vi "测试中.vi"(6 "测试数据":dbl[][](array[numeric]), 7 "XY图":refnum<vi>, 8 "曲线设置":T1={"X轴数据选择"=enum."设置电压", "Y轴组"=[]}, 10 "错误输入（无错误）":errorcluster) -> (2 "错误输出":errorcluster)   [LabVIEW 2021]
uses:
  <vilib>/Utility/miscctls.llb/LVCursorListTypeDef.ctl
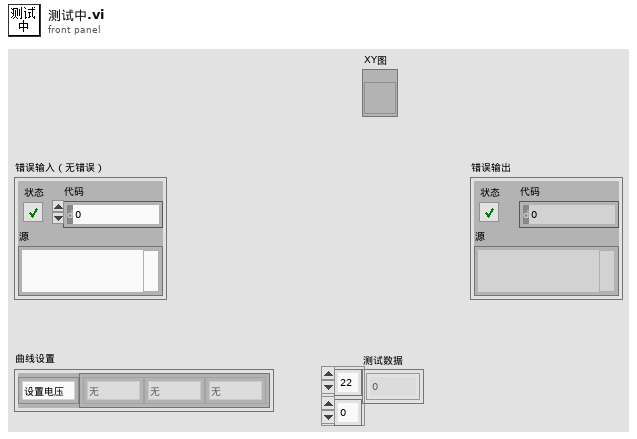
[diagram p1: front panel]
types:
  T1 = typedef "曲线设置.ctl" = cluster{"X轴数据选择":enum16{"时间", "设置电压", "读取电流", "读取电压"}, "Y轴组":enum16{"时间", "设置电压", "读取电流", "读取电压", "无"}[]}
  T2 = typedef "LVCursorListTypeDef.ctl" = cluster{"Name":string, "Color":u32, "Style":u8, "Point Style":u8, "Name Visible":bool, "Allow Drag":bool, "Cursor Mode":u32, "Plot":i32, "Index":i32, "Position":cluster{"X":dbl, "Y":dbl}, "X Scale":u32, "Y Scale":u32, "Watch Plots":i32[], "Watch All Plots":bool, "Plot Area":i32, "Label Offset":cluster{"X":dbl, "Y":dbl}}[]
  T3 = typedef "曲线属性.ctl" = cluster{"曲线名":string, "曲线颜色":u32}
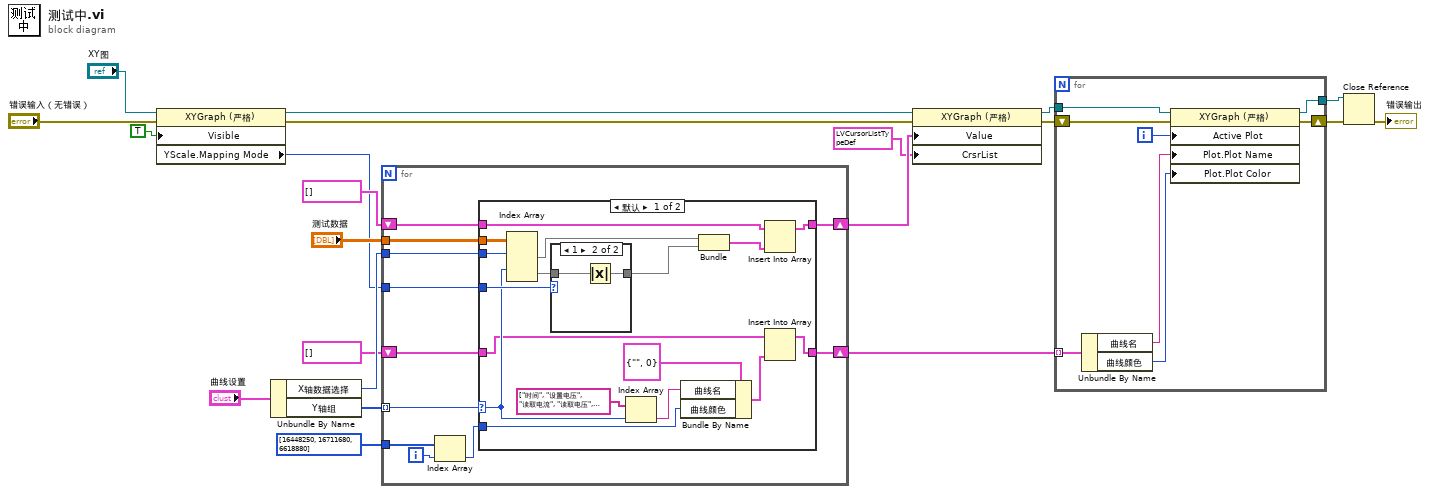
[diagram p0: block diagram]
diagram:
  n1 = property class="XYGraph (严格)"(reference="XY图", error in="错误输入（无错误）", "Visible"=TRUE ("可见")) -> (reference out=w13:refnum<vi>, error out=w14:errorcluster, "YScale.Mapping Mode"=w4:u8)
  n2 = Unbundle By Name("曲线设置") -> ("X轴数据选择"=w18:enum16{"时间", "设置电压", "读取电流", "读取电压"}, "Y轴组"=w17:enum16{"时间", "设置电压", "读取电流", "读取电压", "无"}[])
  n3 = for {
    tunnel: w17 -> [w29] mode=indexing
    tunnel: "测试数据" -> [w32]
    tunnel: w18 -> [w31]
    tunnel: u32[] [16448250, 16711680, 6618880] -> [w23]
    tunnel: w4 -> [w30]
    shift-right: [w27] -> w2
    shift-left: cluster{"测试数据":dbl[], "测试数据":dbl[]}[] [] -> [w28]
    shift-right: [w25] -> w12
    shift-left: cluster{"曲线名":string, "曲线颜色":u32}[] [] -> [w26]
    i -> [w24]
    n4 = Index Array(array=w23, index=w24) -> (element=w22:u32)
    n5 = case shown="默认" w29 {
      selector: w29 -> [w40 _]
      tunnel: w32 -> [w49 _]
      tunnel: w31 -> [w47 _]
      tunnel: w22 -> [w46 _]
      tunnel: w30 -> [w45 _]
      tunnel: w28 -> [w39 w54]
      tunnel: [w37 w54] -> w27
      tunnel: w26 -> [w36 w53]
      tunnel: [w34 w53] -> w25
      frame Default {
        n6 = Index Array(array=w49, index (row) #1=w47, index (row) #2=w40) -> (element #1=w48:dbl[], element #2=w44:dbl[])  [unwired: 2 in]
        n7 = case shown="1" w45 {
          tunnel: w44 -> [w50 w52]
          tunnel: [w50 w51] -> w43
          frame 0, Default {
          }
          frame 1 {
            n8 = Absolute Value(x=w52) -> (abs(x)=w51:dbl[])
          }
        }
        n9 = Index Array(array=string[] ["时间", "设置电压", "读取电流", "读取电压", "无"] ("字符串[]"), index=w40) -> (element=w41:string)
        n10 = Bundle By Name(cluster=T3 {"曲线名"="", "曲线颜色"=0} ("曲线属性"), "曲线名"=w41, "曲线颜色"=w46) -> (w35:T3)
        n11 = Bundle("测试数据"=w48, "测试数据"=w43) -> (w38:cluster{"测试数据":dbl[], "测试数据":dbl[]})  [unwired: 1 in]
        n12 = Insert Into Array(array=w39, new element=w38) -> (w37:cluster{"测试数据":dbl[], "测试数据":dbl[]}[])  [unwired: 1 in]
        n13 = Insert Into Array(array=w36, new element=w35) -> (w34:cluster{"曲线名":string, "曲线颜色":u32}[])  [unwired: 1 in]
      }
      frame "无" {
      }
    }
  }
  n14 = property class="XYGraph (严格)"(reference=w13, error in=w14, "Value"=w2, "CrsrList"=T2 [{"Name"="", "Color"=16776960, "Style"=2, "Point Style"=13, "Name Visible"=FALSE, "Allow Drag"=TRUE, "Cursor Mode"=2, "Plot"=-1, "Index"=0, "Position"={"X"=1.0, "Y"=0.0}, "X Scale"=0, "Y Scale"=0, "Watch Plots"=[], "Watch All Plots"=TRUE, "Plot Area"=0, "Label Offset"={"X"=0.0, "Y"=0.0}}] ("游标列表")) -> (reference out=w11:refnum<vi>, error out=w10:errorcluster)
  n15 = for {
    shift-right: [w61] -> w9
    shift-left: w10 -> [w62]
    tunnel: w12 -> [w55] mode=indexing
    tunnel: w11 -> [w60]
    tunnel: [w59] -> w8
    i -> [w56]
    n16 = Unbundle By Name(w55) -> ("曲线名"=w58:string, "曲线颜色"=w57:u32)
    n17 = property on="属性节点" class="XYGraph (严格)"(reference=w60, error in=w62, "Active Plot"=w56, "Plot.Plot Name"=w58, "Plot.Plot Color"=w57) -> (reference out=w59:refnum<vi>, error out=w61:errorcluster)
  }
  n18 = Close Reference(reference=w8, error in (no error)=w9) -> (error out=→"错误输出":errorcluster)
